vi "midi_ParseDeltaTime.vi"(0 "string":string, 11 "error in (no error)":errorcluster) -> (4 "result string":string, 8 "delta time (tics)":u32, 10 "bytes read":i32, 15 "error out":errorcluster)   [LabVIEW 2013]
doc: "Parse a string of up to four bytes as a delta time, and return the number of tics as an integer."
panel:
  # "midi_ParseDeltaTime"
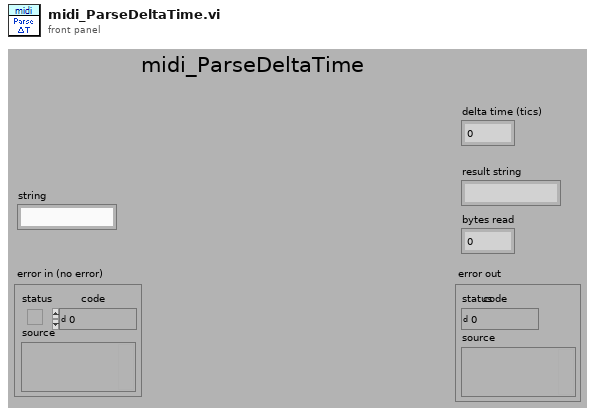
[diagram p1: front panel]
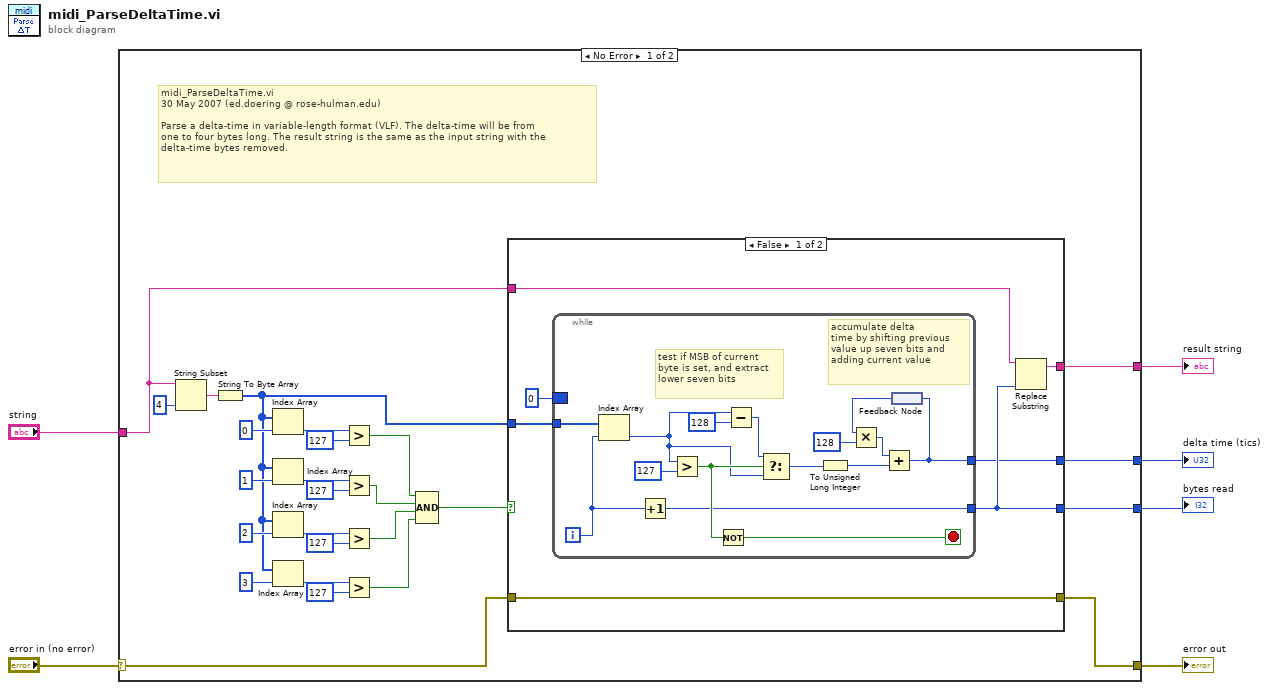
[diagram p0: block diagram]
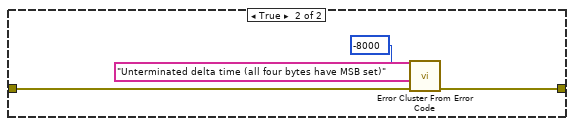
[diagram p2: hidden frame]
diagram:
  n1 = case shown="No Error" "error in (no error)" {
    selector: "error in (no error)" -> [w13 w59]
    tunnel: [w12 w59] -> w5
    tunnel: "string" -> [w7 _]
    tunnel: [w10 _] -> w3
    tunnel: [w9 _] -> w2
    tunnel: [w8 _] -> w1
    frame No Error {
      # "midi_ParseDeltaTime.vi\n30 May 2007 (ed.doering @ rose-hulman.edu)\n\nParse a delta-time in variable-length format (VLF). The delta-time will be from\none to four bytes long. The result string is the same as the input string with the\ndelta-time bytes removed."
      n2 = String Subset(string=w7, length (rest)=4 ("length (rest)")) -> (substring=w31:string)  [unwired: 1 in]
      n3 = String To Byte Array(string=w31) -> (unsigned byte array=w11:u8[])
      n4 = Index Array(array=w11, index=0) -> (element=w29:u8)
      n5 = Index Array(array=w11, index=1) -> (element=w21:u8)
      n6 = Index Array(array=w11, index=2) -> (element=w20:u8)
      n7 = Index Array(array=w11, index=3) -> (element=w19:u8)
      n8 = Greater?(x=w29, y=u8 127) -> (0:w18:bool)
      n9 = Greater?(x=w21, y=u8 127) -> (0:w17:bool)
      n10 = Greater?(x=w20, y=u8 127) -> (0:w16:bool)
      n11 = Greater?(x=w19, y=u8 127) -> (0:w15:bool)
      n12 = Compound Arithmetic op=AND(w18, w17, w16, w15) -> (w14:bool)
      n13 = case shown="False" w14 {
        tunnel: w13 -> [w39 w56]
        tunnel: [w39 w55] -> w12
        tunnel: w11 -> [w37 _]
        tunnel: [w36 _] -> w10
        tunnel: [w35 _] -> w9
        tunnel: [w34 _] -> w8
        tunnel: w7 -> [w33 _]
        frame False {
          n14 = while {
            tunnel: [w51] -> w35
            tunnel: [w46] -> w36
            tunnel: w37 -> [w41]
            border: u32 0 -> [_]
            i -> [w43]
            stop <- w42 stop-if-true
            # "accumulate delta\ntime by shifting previous\nvalue up seven bits and\nadding current value"
            # "test if MSB of current\nbyte is set, and extract\nlower seven bits"
            n15 = Index Array(array=w41, index=w43) -> (element=w40:u8)
            n16 = Increment(x=w43) -> (x+1=w46:i32)
            n17 = Greater?(x=w40, y=u8 127) -> (0:w47:bool)
            n18 = Not(x=w47) -> (.not. x?=w42:bool)
            n19 = Subtract(x=w40, y=u8 128) -> (x-y=w52:u8)
            n20 = Select(t=w52, s=w47, f=w40) -> (s? t:f=w45:u8)
            n21 = To Unsigned Long Integer(number=w45) -> (unsigned 32bit integer=w44:u32)
            n22 = feedback #1() -> (w50:u32)
            n23 = Multiply(x=w50, y=u32 128) -> (x*y=w48:u32)
            n24 = Add(x=w48, y=w44) -> (x+y=w51:u32)
            n25 = feedback-in #1(w51) -> ()
          }
          n26 = Replace Substring(2:w36, 5:w33) -> (1:w34:string)  [unwired: 2 in, 1 out]
        }
        frame True {
          n27 = call <vilib>:"Error Cluster From Error Code.vi"("error in (no error)"=w56, "error message (\"\")"="Unterminated delta time (all four bytes have MSB set)" ("error message (\"\")"), "error code (0)"=-8000) -> ("error out"=w55:errorcluster)  [unwired: 6 in]
        }
      }
    }
    frame Error {
    }
  }
  "error out" <- w5
  "delta time (tics)" <- w2
  "result string" <- w1
  "bytes read" <- w3
